vi "standard frame scan geometry_MD.vi"() -> (3 "frame scan geometry out":waveform(dbl)[](array[waveform]))   [LabVIEW 2012]
uses:
  GFG/GFGnumericGet.vi
  GFG/GFGbooleanGet.vi
  <vilib>/Analysis/coordinate.llb/2D Cartesian Coordinate Rotation (Array).vi
  GFG/GFG library.lvlib
  <vilib>/Analysis/NI_AALPro.lvlib
panel:
  out "x waveform":waveform(dbl)
  out "y waveform":waveform(dbl)
  out "Waveform Graph 2":waveform(dbl)(graph)
  out "Waveform Graph":waveform(dbl)(graph)
  out "y waveform (two frames)":dbl[](array[numeric])
  out "x waveform (two frames)":dbl[](array[numeric])
  out "XY Graph":cluster{"Y":dbl[], "Y":dbl[]}[](graph)
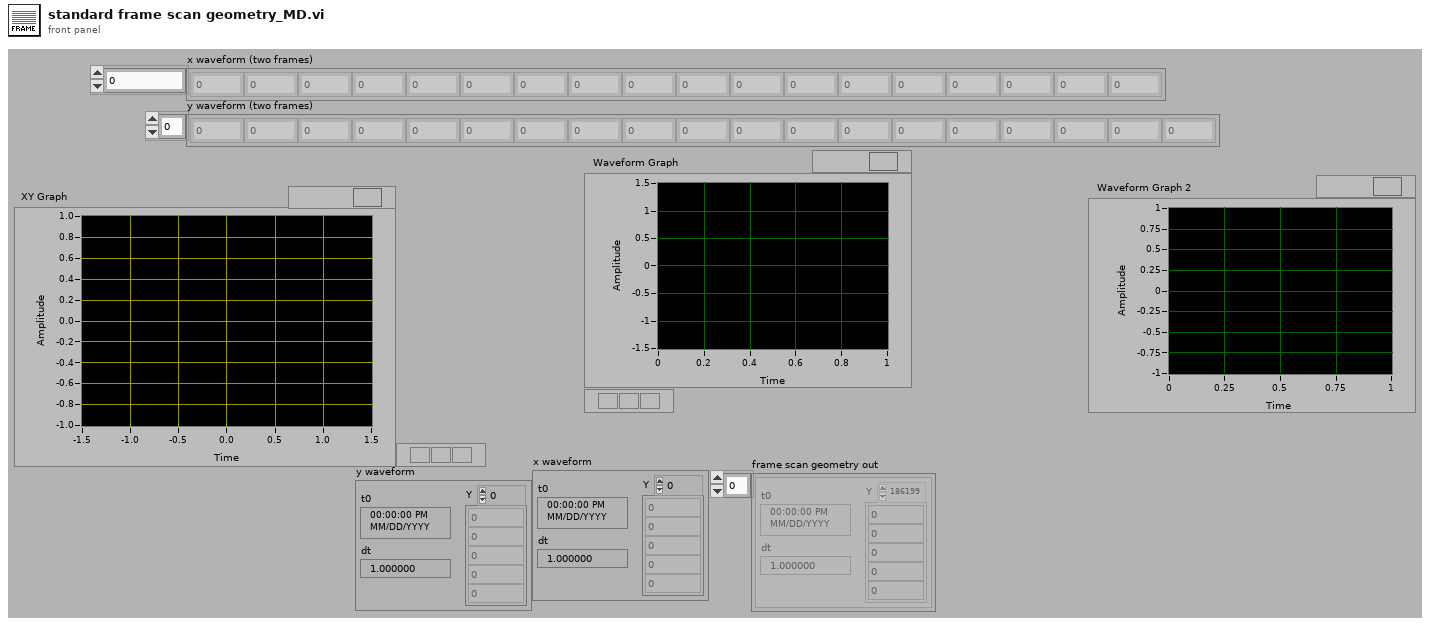
[diagram p1: front panel]
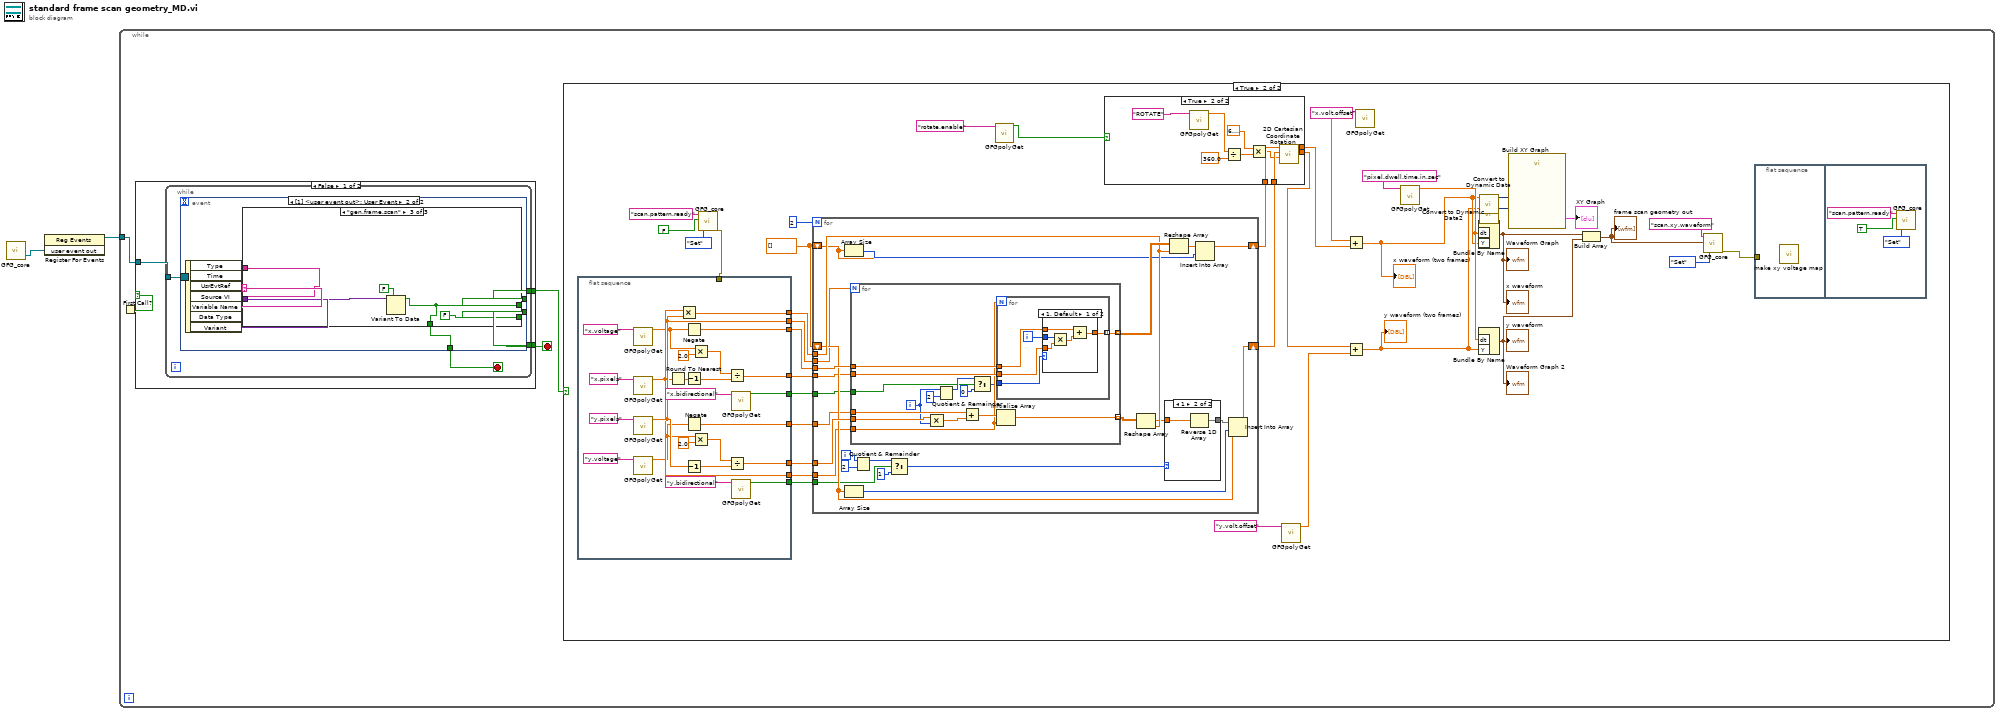
[diagram p0: block diagram]
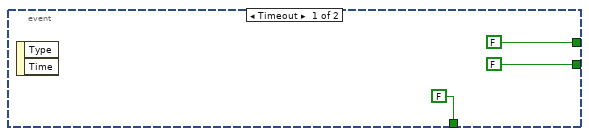
[diagram p2: hidden frame]
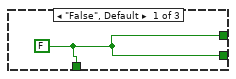
[diagram p3: hidden frame]
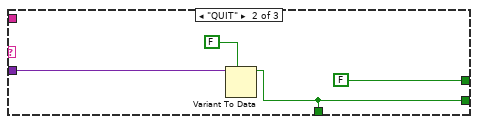
[diagram p4: hidden frame]
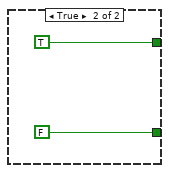
[diagram p5: hidden frame]
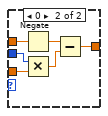
[diagram p9: hidden frame]
diagram:
  n1 = call "GFG_core.vi"() -> ("user event out"=w2:refnum<user-event>)  [unwired: 13 in, 6 out]
  n2 = register-events(w2) -> (reference out=w1:refnum<event-registration>)  [unwired: 2 in, 1 out]
  n3 = while {
    tunnel: w1 -> [w6]
    stop <- w5 stop-if-true
    n4 = First Call?() -> (First Call?: T/F=w3:bool)
    n5 = case shown="False" w3 {
      tunnel: w6 -> [w9 _]
      tunnel: [w8 FALSE ("NewVal")] -> w5
      tunnel: [w7 TRUE ("NewVal")] -> w4
      frame False {
        n6 = while {
          tunnel: w9 -> [w13]
          tunnel: [w11] -> w8
          tunnel: [w12] -> w7
          stop <- w10 stop-if-true
          n7 = event shown="[1] <user event out>: User Event" {
            selector: w13 -> [_ _]
            dyn-events: _ -> [_ _]
            timeout: _ -> [_ _]
            tunnel: [FALSE ("NewVal") w21] -> w12
            tunnel: [FALSE ("NewVal") w20] -> w11
            tunnel: [FALSE w18] -> w10
            event Timeout {
              n8 = event-data() -> ()  [unwired: 1 in, 2 out]
            }
            event User Event {
              n9 = event-data() -> ("Source VI"=w17:string, "Variable Name"=w22:string, "Variant"=w19:variant)  [unwired: 1 in, 4 out]
              n10 = case shown="\"gen.frame.scan\"" w22 {
                tunnel: [w23 FALSE ("NewVal") w28] -> w21
                tunnel: [w23 w24 FALSE] -> w20
                tunnel: w19 -> [_ w27 w29]
                tunnel: [w23 w24 w28] -> w18
                tunnel: w17 -> [_ _ _]
                frame "False", Default {
                  w23 = FALSE ("NewVal")
                }
                frame "QUIT" {
                  n11 = Variant To Data(type=FALSE ("NewVal"), Variant=w27) -> (data=w24:bool)  [unwired: 1 in, 1 out]
                }
                frame "gen.frame.scan" {
                  n12 = Variant To Data(type=FALSE ("NewVal"), Variant=w29) -> (data=w28:bool)  [unwired: 1 in, 1 out]
                }
              }
            }
          }
        }
      }
      frame True {
      }
    }
    n13 = case shown="True" w4 {
      frame False {
      }
      frame True {
        w65 = dbl[] []
        n14 = flat-sequence {
          tunnel: [w93] -> w71
          tunnel: [w92] -> w70
          tunnel: [w90] -> w64
          tunnel: [w86] -> w63
          tunnel: [w85] -> w62
          tunnel: [w84] -> w61
          tunnel: [w82] -> w60
          tunnel: [w76] -> w59
          tunnel: [w74] -> w58
          tunnel: w34 -> [_]
          frame #0 {
            n15 = call-poly "GFGpolyGet.vi"("Variable Name in"="x.voltage" ("Tag in")) -> ("Numeric"=w80:dbl)  [unwired: 9 in, 1 out]
            n16 = call-poly "GFGpolyGet.vi"("Variable Name in"="x.pixels" ("Tag in")) -> ("Numeric"=w82:dbl)  [unwired: 9 in, 1 out]
            n17 = call-poly "GFGpolyGet.vi"("Variable Name in"="y.pixels" ("Tag in")) -> ("Numeric"=w84:dbl)  [unwired: 9 in, 1 out]
            n18 = call-poly "GFGpolyGet.vi"("Variable Name in"="y.voltage" ("Tag in")) -> ("Numeric"=w78:dbl)  [unwired: 9 in, 1 out]
            n19 = Round To Nearest(number=w82) -> (nearest integer value=w72:dbl)
            n20 = Multiply(x=w82, y=w84) -> (x*y=w85:dbl)
            n21 = Negate(x=w80) -> (-x=w93:dbl)
            n22 = Decrement(x=w72) -> (x-1=w89:dbl)
            n23 = Negate(x=w78) -> (-x=w90:dbl)
            n24 = Decrement(x=w84) -> (x-1=w91:dbl)
            n25 = Multiply(x=w80, y=2.0) -> (x*y=w88:dbl)
            n26 = Multiply(x=w78, y=2.0) -> (x*y=w94:dbl)
            n27 = Divide(x=w88, y=w89) -> (x/y=w86:dbl)
            n28 = Divide(x=w94, y=w91) -> (x/y=w92:dbl)
            n29 = call-poly "GFGpolyGet.vi"("Variable Name in"="x.bidirectional" ("Tag in")) -> ("Boolean"=w74:bool)  [unwired: 10 in]
            n30 = call-poly "GFGpolyGet.vi"("Variable Name in"="y.bidirectional" ("Tag in")) -> ("Boolean"=w76:bool)  [unwired: 10 in]
          }
        }
        n31 = call "GFG_core.vi"("Variable Name in"="scan.pattern.ready", "Variant in"=FALSE, "Action"=enum16{"Init", "Set", "Get"}."Set") -> ("error out"=w34:errorcluster)  [unwired: 10 in, 6 out]
        n32 = for {
          N: 2 -> [_]
          tunnel: w71 -> [w135]
          tunnel: w70 -> [w134]
          tunnel: w61 -> [w117]
          tunnel: w62 -> [w131]
          shift-right: [w125] -> w43
          shift-left: w65 -> [w127]
          shift-right: [w121] -> w42
          shift-left: w65 -> [w123]
          tunnel: w60 -> [w120]
          tunnel: w64 -> [w119]
          tunnel: w63 -> [w118]
          tunnel: w59 -> [w112]
          tunnel: w58 -> [w111]
          i -> [w130]
          n33 = Array Size(array=w127) -> (size(s)=w128:i32)
          n34 = Array Size(array=w123) -> (size(s)=w122:i32)
          n35 = for {
            N: w117 -> [_]
            tunnel: w120 -> [w145]
            tunnel: w135 -> [w147]
            tunnel: w134 -> [w153]
            tunnel: [w150] -> w133 mode=indexing
            tunnel: [w149] -> w132 mode=indexing
            tunnel: w119 -> [w148]
            tunnel: w118 -> [w146]
            tunnel: w111 -> [w139]
            i -> [w141]
            n36 = Multiply(x=w153, y=w141) -> (x*y=w152:dbl)
            n37 = Quotient & Remainder(x=w141, y=2) -> (x-y*floor(x/y)=w144:i32)  [unwired: 1 out]
            n38 = Add(x=w148, y=w152) -> (x+y=w151:dbl)
            n39 = Select(t=w144, s=w139, f=0) -> (s? t:f=w140:i32)
            n40 = for {
              N: w145 -> [_]
              tunnel: w146 -> [w158]
              tunnel: [w157] -> w150 mode=indexing
              tunnel: w147 -> [w156]
              tunnel: w140 -> [w154]
              i -> [w155]
              n41 = case shown="1, Default" w154 {
                tunnel: w158 -> [w163 w169]
                tunnel: [w162 w168] -> w157
                tunnel: w156 -> [w161 w167]
                tunnel: w155 -> [w159 w165]
                frame 1, Default {
                  n42 = Multiply(x=w159, y=w163) -> (x*y=w160:dbl)
                  n43 = Add(x=w161, y=w160) -> (x+y=w162:dbl)
                }
                frame 0 {
                  n44 = Negate(x=w167) -> (-x=w164:dbl)
                  n45 = Multiply(x=w165, y=w169) -> (x*y=w166:dbl)
                  n46 = Subtract(x=w164, y=w166) -> (x-y=w168:dbl)
                }
              }
            }
            n47 = Initialize Array(w151, w145) -> (w149:dbl[])
          }
          n48 = Quotient & Remainder(x=w130, y=2) -> (x-y*floor(x/y)=w114:i32)  [unwired: 1 out]
          n49 = Select(t=w114, s=w112, f=1) -> (s? t:f=w113:i32)
          n50 = Reshape Array(w132, w131) -> (w129:dbl[])
          n51 = case shown="1" w113 {
            tunnel: [w136 w137] -> w124
            tunnel: w129 -> [w136 w138]
            frame 0, Default {
            }
            frame 1 {
              n52 = Reverse 1D Array(array=w138) -> (reversed array=w137:dbl[])
            }
          }
          n53 = Reshape Array(w133, w131) -> (w126:dbl[])
          n54 = Insert Into Array(array=w126, index=w128, new element=w127) -> (w125:dbl[])
          n55 = Insert Into Array(array=w124, index=w122, new element=w123) -> (w121:dbl[])
        }
        n56 = call-poly "GFGpolyGet.vi"("Variable Name in"="rotate.enable" ("Tag in")) -> ("Boolean"=w45:bool)  [unwired: 10 in]
        n57 = case shown="True" w45 {
          tunnel: w43 -> [w99 w110]
          tunnel: w42 -> [w100 w109]
          tunnel: [w99 w102] -> w41
          tunnel: [w100 w101] -> w40
          frame False {
          }
          frame True {
            n58 = call-poly "GFGpolyGet.vi"("Variable Name in"="ROTATE" ("Tag in")) -> ("Numeric"=w104:dbl)  [unwired: 9 in, 1 out]
            n59 = Divide(x=w104, y=360.0) -> (x/y=w105:dbl)
            n60 = Multiply(x=6.283185307179586, y=w105) -> (x*y=w103:dbl)
            n61 = call-poly <vilib>:"2D Cartesian Coordinate Rotation.vi"("theta"=w103, "Y"=w109, "X"=w110) -> ("Y Out"=w101:dbl[], "X Out"=w102:dbl[])  [unwired: 6 in, 1 out]
          }
        }
        n62 = call-poly "GFGpolyGet.vi"("Variable Name in"="y.volt.offset" ("Tag in")) -> ("Numeric"=w53:dbl)  [unwired: 9 in, 1 out]
        n63 = Add(x=w40, y=w53) -> (x+y=w38:dbl[])
        "y waveform (two frames)" <- w38
        n64 = call-poly "GFGpolyGet.vi"("Variable Name in"="x.volt.offset" ("Tag in")) -> ("Numeric"=w55:dbl)  [unwired: 9 in, 1 out]
        n65 = Add(x=w55, y=w41) -> (x+y=w39:dbl[])
        "x waveform (two frames)" <- w39
        n66 = call-poly "GFGpolyGet.vi"("Variable Name in"="pixel.dwell.time.in.sec" ("Tag in")) -> ("Numeric"=w47:dbl)  [unwired: 9 in, 1 out]
        n67 = Bundle By Name("dt"=w47, "Y"=w39) -> (w52:waveform(dbl))  [unwired: 1 in]
        "Waveform Graph" <- w52
        "x waveform" <- w52
        n68 = Bundle By Name("dt"=w47, "Y"=w38) -> (w51:waveform(dbl))  [unwired: 1 in]
        "Waveform Graph 2" <- w51
        "y waveform" <- w51
        n69 = call "Convert to Dynamic Data"("Array"=w39) -> ("Dynamic Data Type"=w68:dynamicdata)  [unwired: 3 in]
        n70 = call "Convert to Dynamic Data2"("Array"=w38) -> ("Dynamic Data Type"=w67:dynamicdata)  [unwired: 3 in]
        n71 = call "Build XY Graph"("Y Input"=w67, "X Input"=w68) -> ("XY Graph"=→"XY Graph":cluster{"Y":dbl[], "Y":dbl[]}[])  [unwired: 8 in, 1 out]
        n72 = Build Array(w52, w51) -> (w49:waveform(dbl)[])
        "frame scan geometry out" <- w49
        n73 = call "GFG_core.vi"("Variable Name in"="scan.xy.waveform", "Variant in"=w49, "Action"=enum16{"Init", "Set", "Get"}."Set") -> ("error out"=w44:errorcluster)  [unwired: 10 in, 6 out]
        n74 = flat-sequence {
          tunnel: w44 -> [_]
          frame #0 {
            n75 = call "make xy voltage map.vi"() -> ()  [unwired: 12 in]
          }
          frame #1 {
            n76 = call "GFG_core.vi"("Variable Name in"="scan.pattern.ready", "Variant in"=TRUE, "Action"=enum16{"Init", "Set", "Get"}."Set") -> ()  [unwired: 10 in, 7 out]
          }
        }
      }
    }
  }
